vi "zmq_socket.vi"(4 "error in":errorcluster, 5 "linger (ms)":i32, 6 "socket type":T1, 7 "context in":refnum<class "zmq_context.lvclass">) -> (0 "error out":errorcluster, 2 "socket out":refnum<class "zmq_socket.lvclass">, 3 "context out":refnum<class "zmq_context.lvclass">)   [LabVIEW 2010, in "zeromq.lvlib" / "zmq_context.lvclass"]
doc: "Create a socket of flavour <b>socket type</b> in context <b>ctx in</b> and linger time <b>linger</b> milliseconds (time permitted after zmq_term to finish queued operations).\n\nNote that ZeroMQ creates sockets with infinite linger (ZMQ_LINGER) by default, which is undesirable in a managed environment like LabVIEW since it hangs the parent process. But set it to -1 should infinite linger be required.\n\nDetailed API documentation: http://api.zeromq.org/3-2:zmq-socket"
uses:
  zmq_context.lvclass
  socket_type.ctl
  zmq_socket.lvclass
  zmq_context.lvclass/zmq_context.ctl
  <vilib>/Utility/error.llb/Error Cluster From Error Code.vi
  zeromq.lvlib
panel:
  # "ØMQ"
  # "labview"
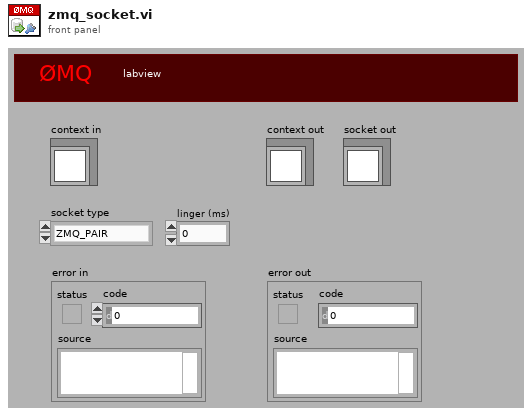
[diagram p1: front panel]
types:
  T1 = typedef "zeromq.lvlib/socket_type.ctl" = enum8{"ZMQ_PAIR", "ZMQ_PUB", "ZMQ_SUB", "ZMQ_REQ", "ZMQ_REP", "ZMQ_DEALER", "ZMQ_ROUTER", "ZMQ_PULL", "ZMQ_PUSH", "ZMQ_XPUB", "ZMQ_XSUB"}
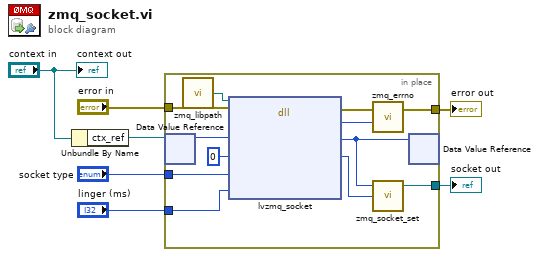
[diagram p0: block diagram]
diagram:
  n1 = Unbundle By Name("context in") -> ("ctx_ref"=w1:refnum<data-value>)
  n2 = in-place {
    in-place-border: "error in" -> [w19]
    in-place-border: "socket type" -> [w18]
    in-place-border: "linger (ms)" -> [w15]
    in-place-border: [w14] -> w3
    in-place-border: [w12] -> w2
    n3 = in-place-dvr #1(w1) -> (w11:u64)  [unwired: 1 out]
    n4 = call "zmq_libpath.vi"() -> ("path"=w8:path)
    n5 = dll-call lib="?" fn="lvzmq_socket"(path in=w8, error in=w19, "ctx_obj"=w11, "sock_obj"=u64 0, "type"=w18, "linger"=w15) -> (error out=w17:errorcluster, "return type"=w16:i32, "ctx_obj"=w10:u64, "sock_obj"=w13:u64)  [unwired: 3 in, 1 out]
    n6 = call "zmq_errno.vi"("retval"=w16, "error in"=w17) -> ("error out"=w14:errorcluster)  [unwired: 1 out]
    n7 = call "zmq_socket_set.vi"("socket"=w13, "context"=w10) -> ("socket out"=w12:refnum<class "zmq_socket.lvclass">)  [unwired: 2 in, 1 out]
    n8 = in-place-dvr #1(w10) -> ()  [unwired: 2 out]
  }
  "error out" <- w3
  "socket out" <- w2
  "context out" <- "context in"
